vi "Set Double Data.vi"(8 "error in (no error)":errorcluster, 9 "Value":dbl, 10 "Name":string, 11 "DoubleDictionary in":refnum<class "DoubleDictionary.lvclass">) -> (0 "error out":errorcluster, 3 "DoubleDictionary out":refnum<class "DoubleDictionary.lvclass">)   [LabVIEW 2014, in "bmlv.lvlib" / "DoubleDictionary.lvclass"]
uses:
  DoubleDictionary.lvclass
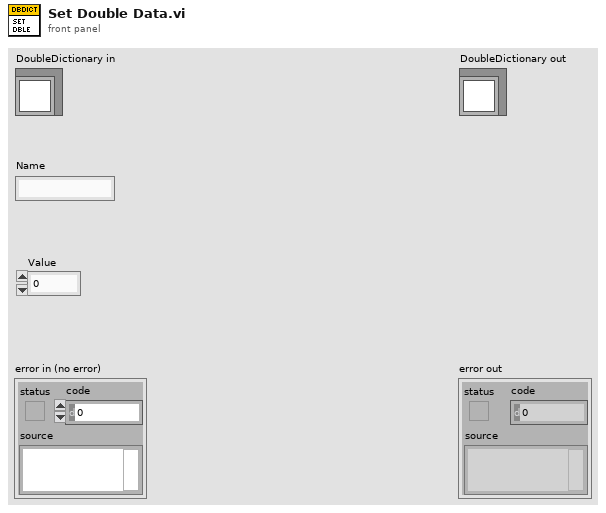
[diagram p1: front panel]
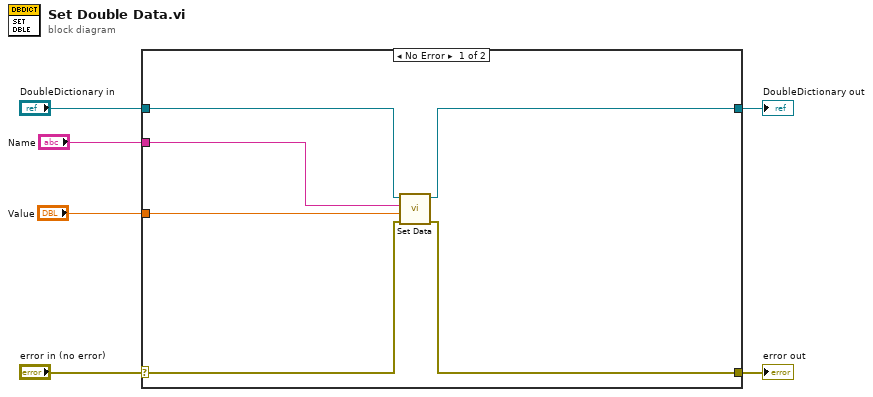
[diagram p0: block diagram]
diagram:
  n1 = case shown="No Error" "error in (no error)" {
    selector: "error in (no error)" -> [w11 w14]
    tunnel: [w10 w14] -> w5
    tunnel: [w8 w13] -> w3
    tunnel: "DoubleDictionary in" -> [w9 w13]
    tunnel: "Value" -> [w12 _]
    tunnel: "Name" -> [w7 _]
    frame No Error {
      n2 = call-dynamic "Set Data.vi"("error in (no error)"=w11, "Data"=w12, "Name"=w7, "Dictionary in"=w9) -> ("error out"=w10:errorcluster, "Dictionary out"=w8:refnum<class "DoubleDictionary.lvclass">)  [unwired: 6 in]
    }
    frame Error {
    }
  }
  "error out" <- w5
  "DoubleDictionary out" <- w3
